vi "marshalling.vi"(8 "error in (no error)":errorcluster, 10 "Variant":variant, 11 "Serializer in":refnum<class "Serializer.JKI-JSON.lvclass">) -> (0 "error out":errorcluster, 2 "String":string, 3 "Serializer out":refnum<class "Serializer.JKI-JSON.lvclass">)   [LabVIEW 2017, in "Serializer.JKI-JSON.lvclass"]
uses:
  Serializer.JKI-JSON.lvclass
  <vilib>/addons/_JKI.lib/Serialization/JSON/JKI JSON Serialization.lvlib
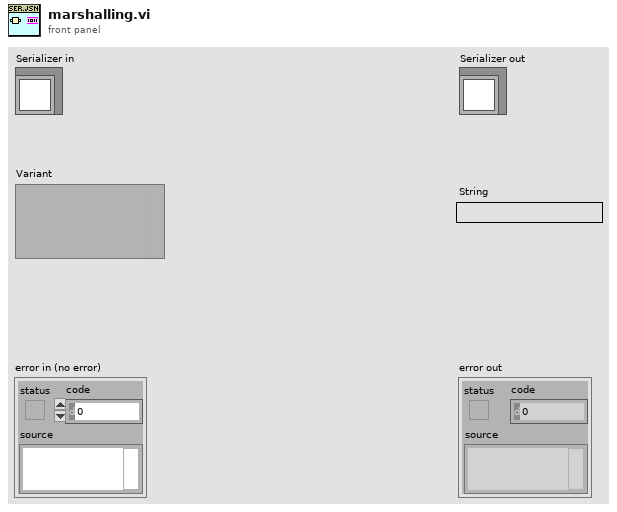
[diagram p1: front panel]
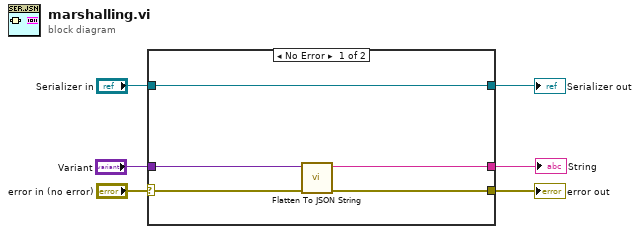
[diagram p0: block diagram]
diagram:
  n1 = case shown="No Error" "error in (no error)" {
    selector: "error in (no error)" -> [w9 w13]
    tunnel: [w8 w13] -> w3
    tunnel: [w11 w12] -> w1
    tunnel: "Serializer in" -> [w11 w12]
    tunnel: "Variant" -> [w10 _]
    tunnel: [w7 _] -> w2
    frame No Error {
      n2 = call <vilib>:"Flatten To JSON String.vi"("error in (no error)"=w9, "Variant"=w10) -> ("error out"=w8:errorcluster, "JSON String"=w7:string)  [unwired: 8 in]
    }
    frame Error {
    }
  }
  "error out" <- w3
  "Serializer out" <- w1
  "String" <- w2
